vi "Hello World!.vi"() -> ()   [LabVIEW 2018]
panel:
  in  "message":string="HELLO WORLD!"
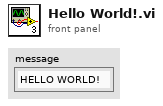
[diagram p1: front panel]
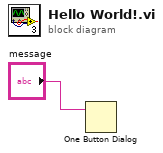
[diagram p0: block diagram]
diagram:
  n1 = One Button Dialog(message="message") -> ()  [unwired: 1 in, 1 out]
